vi "LQR.vi"(2 "DL":dbl[][](array[numeric]), 3 "M":dbl[][](array[numeric]), 4 "R":dbl[][](array[numeric]), 5 "Q":dbl[][](array[numeric])) -> (0 "Kp":dbl[][](array[numeric]), 1 "Kd":dbl[][](array[numeric]))   [LabVIEW 2012]
uses:
  <vilib>/imath/engines/lvmath2/RunTimeEngine/ErrorHandling/NIMS_Finalize Error.vi
  <vilib>/imath/engines/lvmath2/RunTimeEngine/NodeEndStatement/NIMS_NodeEndStatement_Output.vi
  <instcachedir>/0/NIMS_NodeEndStatement_Output_53EC0D466D134D7ABD903AC30B43404B.lvgen/NIMS_NodeEndStatement_Output_53EC0D466D134D7ABD903AC30B43404B_002.vi
  <vilib>/imath/engines/lvmath2/RunTimeEngine/BuiltInFunctions/inv/NIMS_inv(GM).vi
  <instcachedir>/0/NIMS_inv(GM)_A6DF8FE880224208AACFE4CF9F659502.lvgen/NIMS_inv(GM)_A6DF8FE880224208AACFE4CF9F659502_000.vi
  <vilib>/imath/engines/lvmath2/RunTimeEngine/ErrorHandling/NIMS_Error From Error Code.vi
  <vilib>/imath/engines/lvmath2/RunTimeEngine/RowToken/NIMS_RowToken_M_M.vi
  <instcachedir>/0/NIMS_RowToken_M_M_AAD54A35165A48D39931237C063576F0.lvgen/NIMS_RowToken_M_M_AAD54A35165A48D39931237C063576F0_005.vi
  <vilib>/imath/engines/lvmath2/RunTimeEngine/ArithmeticOperatorToken/NIMS_ArithmeticOperator_multmx.vi
  <instcachedir>/0/NIMS_ArithmeticOperator_multmx_B852E135005D4BB784CAAABF10F283E0.lvgen/NIMS_ArithmeticOperator_multmx_B852E135005D4BB784CAAABF10F283E0_004.vi
  <instcachedir>/0/NIMS_RowToken_M_M_AAD54A35165A48D39931237C063576F0.lvgen/NIMS_RowToken_M_M_AAD54A35165A48D39931237C063576F0_004.vi
  <vilib>/imath/engines/lvmath2/RunTimeEngine/MatrixToken/NIMS_MatrixToken_M_M.vi
  <instcachedir>/0/NIMS_MatrixToken_M_M_5BB2FEE2C55E4E95AB6D16A17B4F9783.lvgen/NIMS_MatrixToken_M_M_5BB2FEE2C55E4E95AB6D16A17B4F9783_004.vi
  <vilib>/imath/engines/lvmath2/RunTimeEngine/ErrorHandling/NIMS_Create Error From Enums.vi
  <vilib>/imathl/engines/lvmath/Functions/Error Handling/Create Error.vi
  <vilib>/imath/engines/lvmath/Plug In/Control Design/BuiltInFunctions/lqr/NIMS_CD_lqr(A,B,Q,R,N).vi
  <vilib>/imath/engines/lvmath2/RunTimeEngine/RangeToken/NIMS_Range_R2.vi
  <vilib>/imath/engines/lvmath2/RunTimeEngine/VariableToken/Read/NIMS_Get Elements - SorM($,_) - Check.vi
  <instcachedir>/0/NIMS_Get Elements - SorM($,_) - Check_FA034EA6D1B34B7583DE730A7D862D9F.lvgen/NIMS_Get Elements - SorM($,_) - Check_FA034EA6D1B34B7583DE730A7D862D9F_003.vi
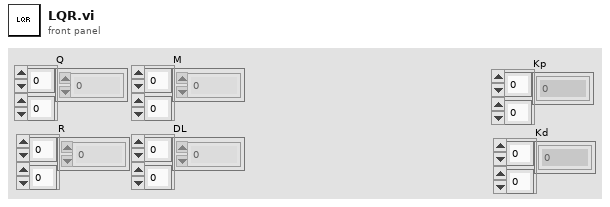
[diagram p1: front panel]
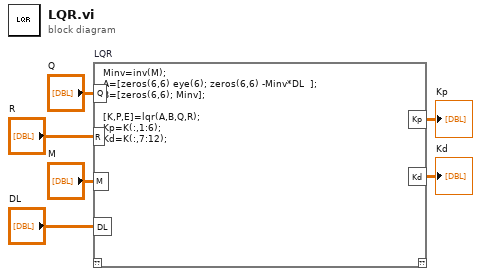
[diagram p0: block diagram]
diagram:
  n1 = mathscript code="Minv=inv(M);\nA=[zeros(6,6) eye(6); zeros(6,6) -Minv*DL  ];\nB=[zeros(6,6); Minv];\n\n[K,P,E]=lqr(A,B,Q,R);\nKp=K(:,1:6);\nKd=K(:,7:12);" "LQR"("Q"="Q", "R"="R", "M"="M", "DL"="DL") -> ("Kp"=→"Kp":dbl[][], "Kd"=→"Kd":dbl[][])  [unwired: 1 in, 1 out]
